vi "DeviceLookupNew.vi"(4 "error in (no error)":errorcluster, 7 "report in":refnum<class "NI_report.lvclass">) -> (0 "error out":errorcluster, 1 "[[Device Types]]":string[][](array[string]), 2 "[[DeviceTypesVals]]":i32[][](array[numeric]), 3 "report out":refnum<class "NI_report.lvclass">)   [LabVIEW 2015]
uses:
  <vilib>/Utility/NIReport.llb/NI_report.lvclass
  <vilib>/addons/_office/excel.llb/Excel Get Data ([str]).vi
  <vilib>/addons/_office/excel.llb/Excel Get Data ([i32]).vi
  <vilib>/addons/_office/NI_ReportGenerationToolkit.lvlib
  <vilib>/Utility/NIReport.llb/Excel/NI_Excel.lvclass
panel:
  out "[[DeviceTypesVals]] 2":i32[][](array[numeric])
  out "[[Device Types]] 2":string[][](array[string])
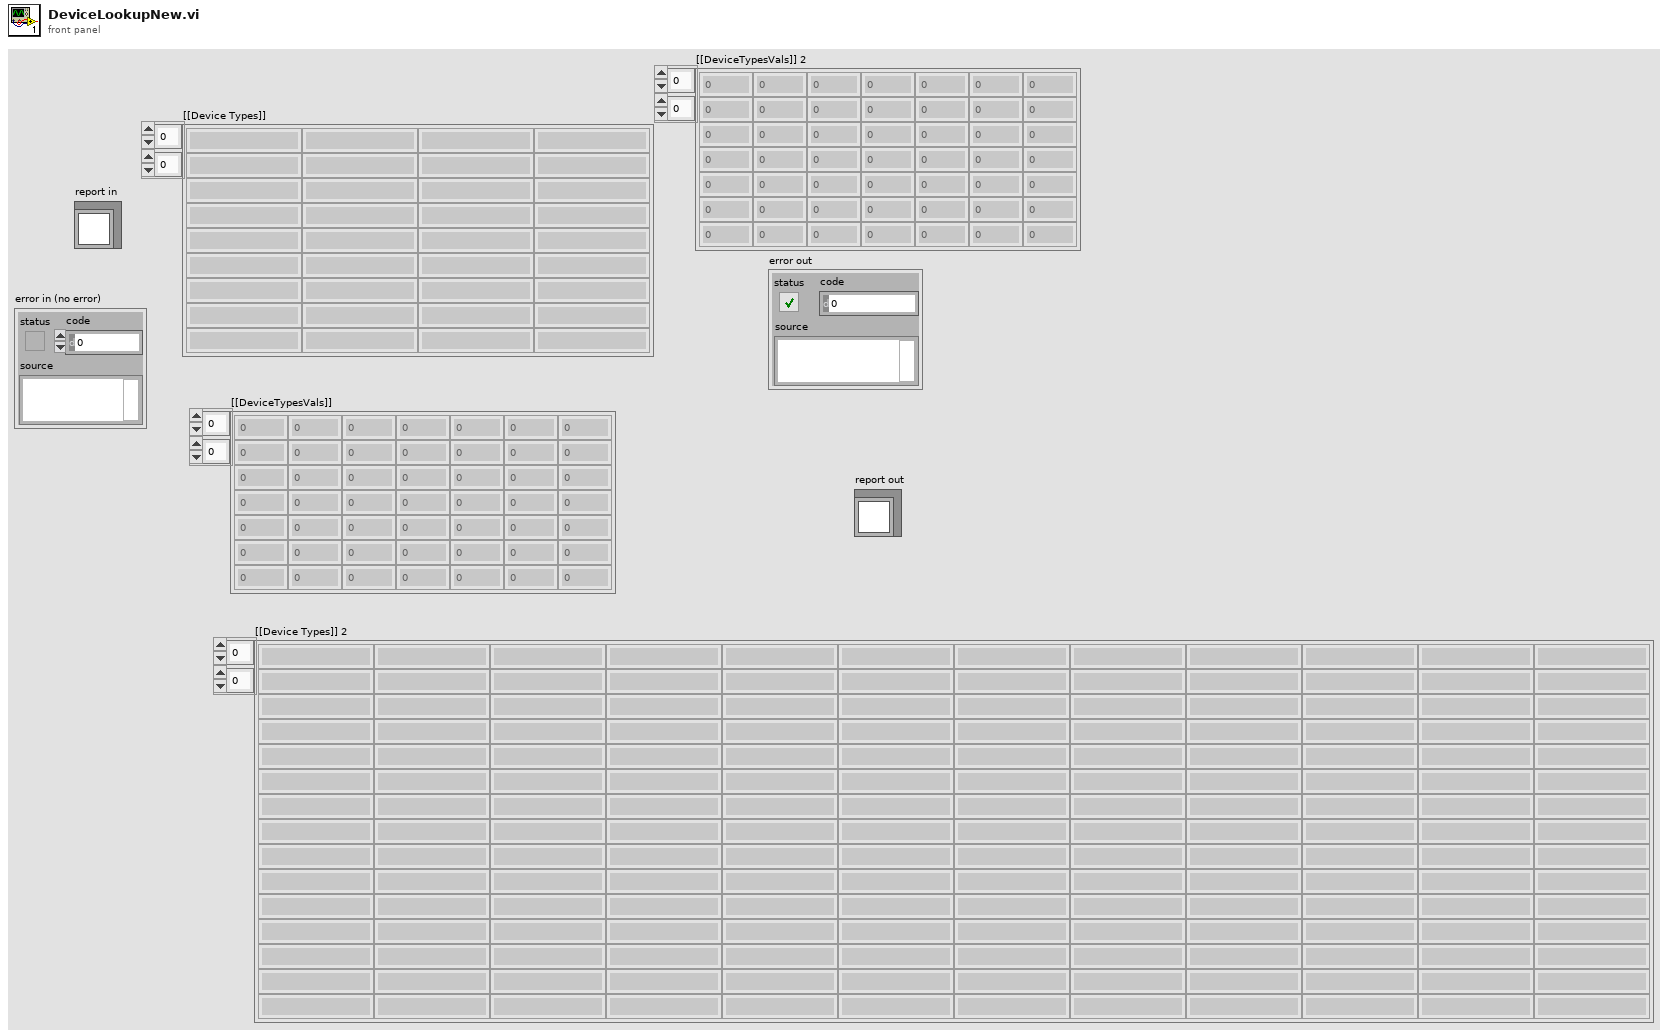
[diagram p1: front panel]
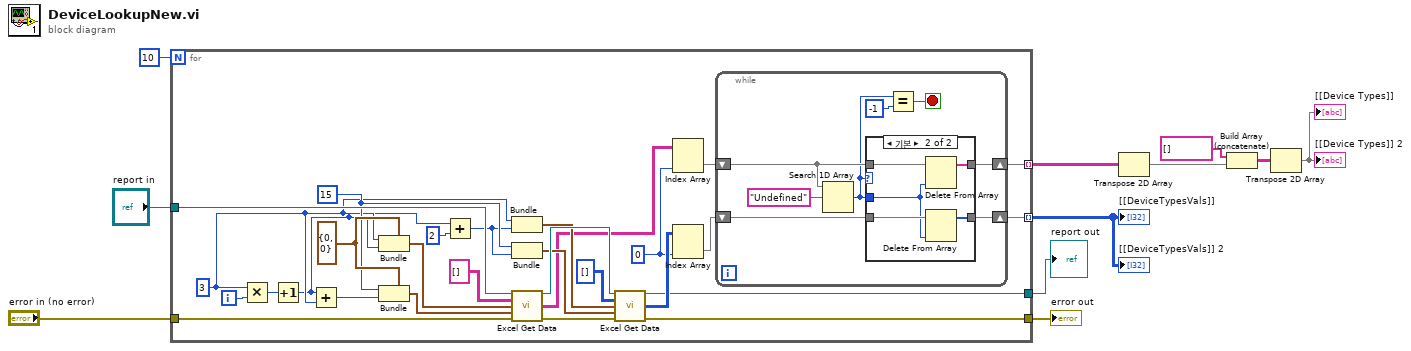
[diagram p0: block diagram]
diagram:
  n1 = for {
    N: 10 -> [_]
    tunnel: "report in" -> [w37]
    tunnel: "error in (no error)" -> [w24]
    tunnel: [w15] -> w8 mode=indexing
    tunnel: [w14] -> w4 mode=indexing
    tunnel: [w13] -> w2
    tunnel: [w12] -> w1
    i -> [w20]
    w21 = 0 ("disabled index (col)")
    w32 = 15 ("row")
    w31 = 3 ("row")
    w36 = cluster{"row":i32, "column":i32} {"row"=0, "column"=0} ("start (-1, -1)")
    n2 = Multiply(x=w31, y=w20) -> (x*y=w19:i32)
    n3 = Increment(x=w19) -> (x+1=w18:i32)
    n4 = Add(x=w18, y=w31) -> (x+y=w29:i32)
    n5 = Bundle(cluster=w36, "row"=w31, "column"=w18) -> (w38:cluster{"row":i32, "column":i32})
    n6 = Bundle(cluster=w36, "row"=w32, "column"=w29) -> (w35:cluster{"row":i32, "column":i32})
    n7 = Add(x=w18, y=2) -> (x+y=w28:i32)
    n8 = Bundle("row"=w31, w28) -> (w27:cluster{"row":i32, i32})  [unwired: 1 in]
    n9 = Bundle("row"=w32, w28) -> (w26:cluster{"row":i32, i32})  [unwired: 1 in]
    n10 = call-poly <vilib>:"Excel Get Data.vi"("report in"=w37, "data type"=string[][] [], "start (-1, -1)"=w38, "end (-1, -1)"=w35, "error in (no error)"=w24) -> ("report out"=w33:refnum<class "NI_report.lvclass">, "data"=w23:string[][], "error out"=w25:errorcluster)  [unwired: 8 in]
    n11 = call-poly <vilib>:"Excel Get Data.vi"("report in"=w33, "data type"=i32[][] [], "start (-1, -1)"=w27, "end (-1, -1)"=w26, "error in (no error)"=w25) -> ("report out"=w13:refnum<class "NI_report.lvclass">, "data"=w22:i32[][], "error out"=w12:errorcluster)  [unwired: 8 in]
    n12 = Index Array(array=w23, index (col)=w21) -> (element=w17:string[])  [unwired: 1 in]
    n13 = Index Array(array=w22, index (col)=w21) -> (element=w16:i32[])  [unwired: 1 in]
    n14 = while {
      shift-right: [w46] -> w14
      shift-left: w17 -> [w43]
      shift-right: [w45] -> w15
      shift-left: w16 -> [w47]
      stop <- w42 stop-if-true
      n15 = Search 1D Array(1D array=w43, element="Undefined") -> (index of element=w40:i32)  [unwired: 1 in]
      n16 = case shown="기본" w40 {
        tunnel: w47 -> [w48 w54]
        tunnel: [w49 w53] -> w46
        tunnel: [w48 w52] -> w45
        tunnel: w40 -> [_ w51]
        tunnel: w43 -> [w49 w50]
        frame -1 {
        }
        frame Default {
          n17 = Delete From Array(array=w50, index=w51) -> (array with subset deleted=w53:string[])  [unwired: 1 in, 1 out]
          n18 = Delete From Array(array=w54, index=w51) -> (array with subset deleted=w52:i32[])  [unwired: 1 in, 1 out]
        }
      }
      n19 = Equal?(x=w40, y=-1) -> (x = y?=w42:bool)
    }
  }
  "[[DeviceTypesVals]]" <- w8
  "report out" <- w2
  "[[DeviceTypesVals]] 2" <- w8
  "error out" <- w1
  n20 = Transpose 2D Array(2D array=w4) -> (transposed array=w7:string[][])
  n21 = Build Array (concatenate)(string[] [] ("element"), w7) -> (w6:string[][])
  n22 = Transpose 2D Array(2D array=w6) -> (transposed array=→"[[Device Types]]" →"[[Device Types]] 2":string[][])
